vi "Periodic Tasks.vi"(8 "error in":errorcluster) -> ()   [LabVIEW 2016]
doc: "This VI runs in parallel to other tasks. It can contain as many user-defined periodic loops as you need. These can carry out PID or other sorts of timed response."
uses:
  <vilib>/Rock Robotics/WPI/Utilities/WPI_GetSetVariantRefNum.vi
  Robot Global Data.vi
  <vilib>/Rock Robotics/Network Tables/NT Write Number.vi
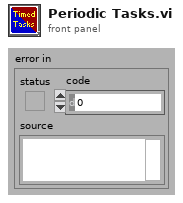
[diagram p1: front panel]
types:
  T1 = typedef "WPI_JoystickDevRef.ctl" = cluster{"Device":T2}
  T2 = typedef "WPI_JoystickDeviceEnum.ctl" = enum16{"USB 0", "USB 1", "USB 2", "USB 3", "USB 4", "USB 5"}
  T3 = typedef "WPI_RobotDriveDevRef.ctl" = cluster{"DevStatus":errorcluster, "Motors[]":T4[], "Square Inputs":bool, "Max Output":dbl}
  T4 = typedef "WPI_MotorControlDeviceRef.ctl" = cluster{"DeviceStatus":errorcluster, "Type":T5, "PWM":cluster{"PWM Channel":T6, "DeadBand":T7}, "CAN":cluster{"Device Number":u8, "SetOutput VI Ref":variant, "GetOutput VI Ref":variant, "Enable VI Ref":variant, "Disable VI Ref":variant, "Data":variant}, "Invert":bool}
  T5 = typedef "WPI_MotorControlType.ctl" = enum16{"PWM", "CAN"}
  T6 = typedef "FPGA_DIOPWMChannel.ctl" = enum8{"PWM 0", "PWM 1", "PWM 2", "PWM 3", "PWM 4", "PWM 5", "PWM 6", "PWM 7", "PWM 8", "PWM 9", "PWM MXP 0", "PWM MXP 1", "PWM MXP 2", "PWM MXP 3", "PWM MXP 4", "PWM MXP 5", "PWM MXP 6", "PWM MXP 7", "PWM MXP 8", "PWM MXP 9", "Invalid"}
  T7 = typedef "WPI_PWMDeadband.ctl" = cluster{"Name":string, "maxPositivePwm":i32, "minPositivePwm":i32, "centerPwm":i32, "maxNegativePwm":i32, "minNegativePwm":i32, "angularRange":u16}
  T8 = typedef "WPI_EncoderDevRef.ctl" = cluster{"DevStatus":errorcluster, "EncoderIndex":T9, "CounterIndex":T10, "DistancePerCount":dbl, "Decoding Type":T11}
  T9 = typedef "FPGA_EncoderIdx.ctl" = enum8{"Enc 0", "Enc 1", "Enc 2", "Enc 3", "Enc 4", "Enc 5", "Enc 6", "Enc 7", "Invalid"}
  T10 = typedef "FPGA_CounterCtrSystemIndex.ctl" = enum8{"Ctr 0", "Ctr 1", "Ctr 2", "Ctr 3", "Ctr 4", "Ctr 5", "Ctr 6", "Ctr 7", "Invalid"}
  T11 = typedef "WPI_EncoderType.ctl" = enum16{"1x", "2x", "4x"}
  T12 = typedef "WPI_ServoDeviceRef.ctl" = cluster{"DeviceStatus":errorcluster, "PWM Channel":T6, "DeadBand":T7}
  T13 = cluster{"JoystickDevRef":T1, "RobotDriveDevRef":T3, "JoystickDevRef":T1}
  T14 = cluster{"Buttons[0]":bool, "Buttons[1]":bool, "Buttons[2]":bool, "Buttons[3]":bool, "Buttons[4]":bool, "Buttons[5]":bool, "Buttons[6]":bool, "Buttons[7]":bool, "Buttons[8]":bool}
  T15 = cluster{"Axes[0]":dbl, "Axes[1]":dbl, "Axes[2]":dbl, "Axes[3]":dbl, "Axes[4]":dbl, "Axes[5]":dbl, "Axes[6]":dbl, "Axes[7]":dbl, "Axes[8]":dbl}
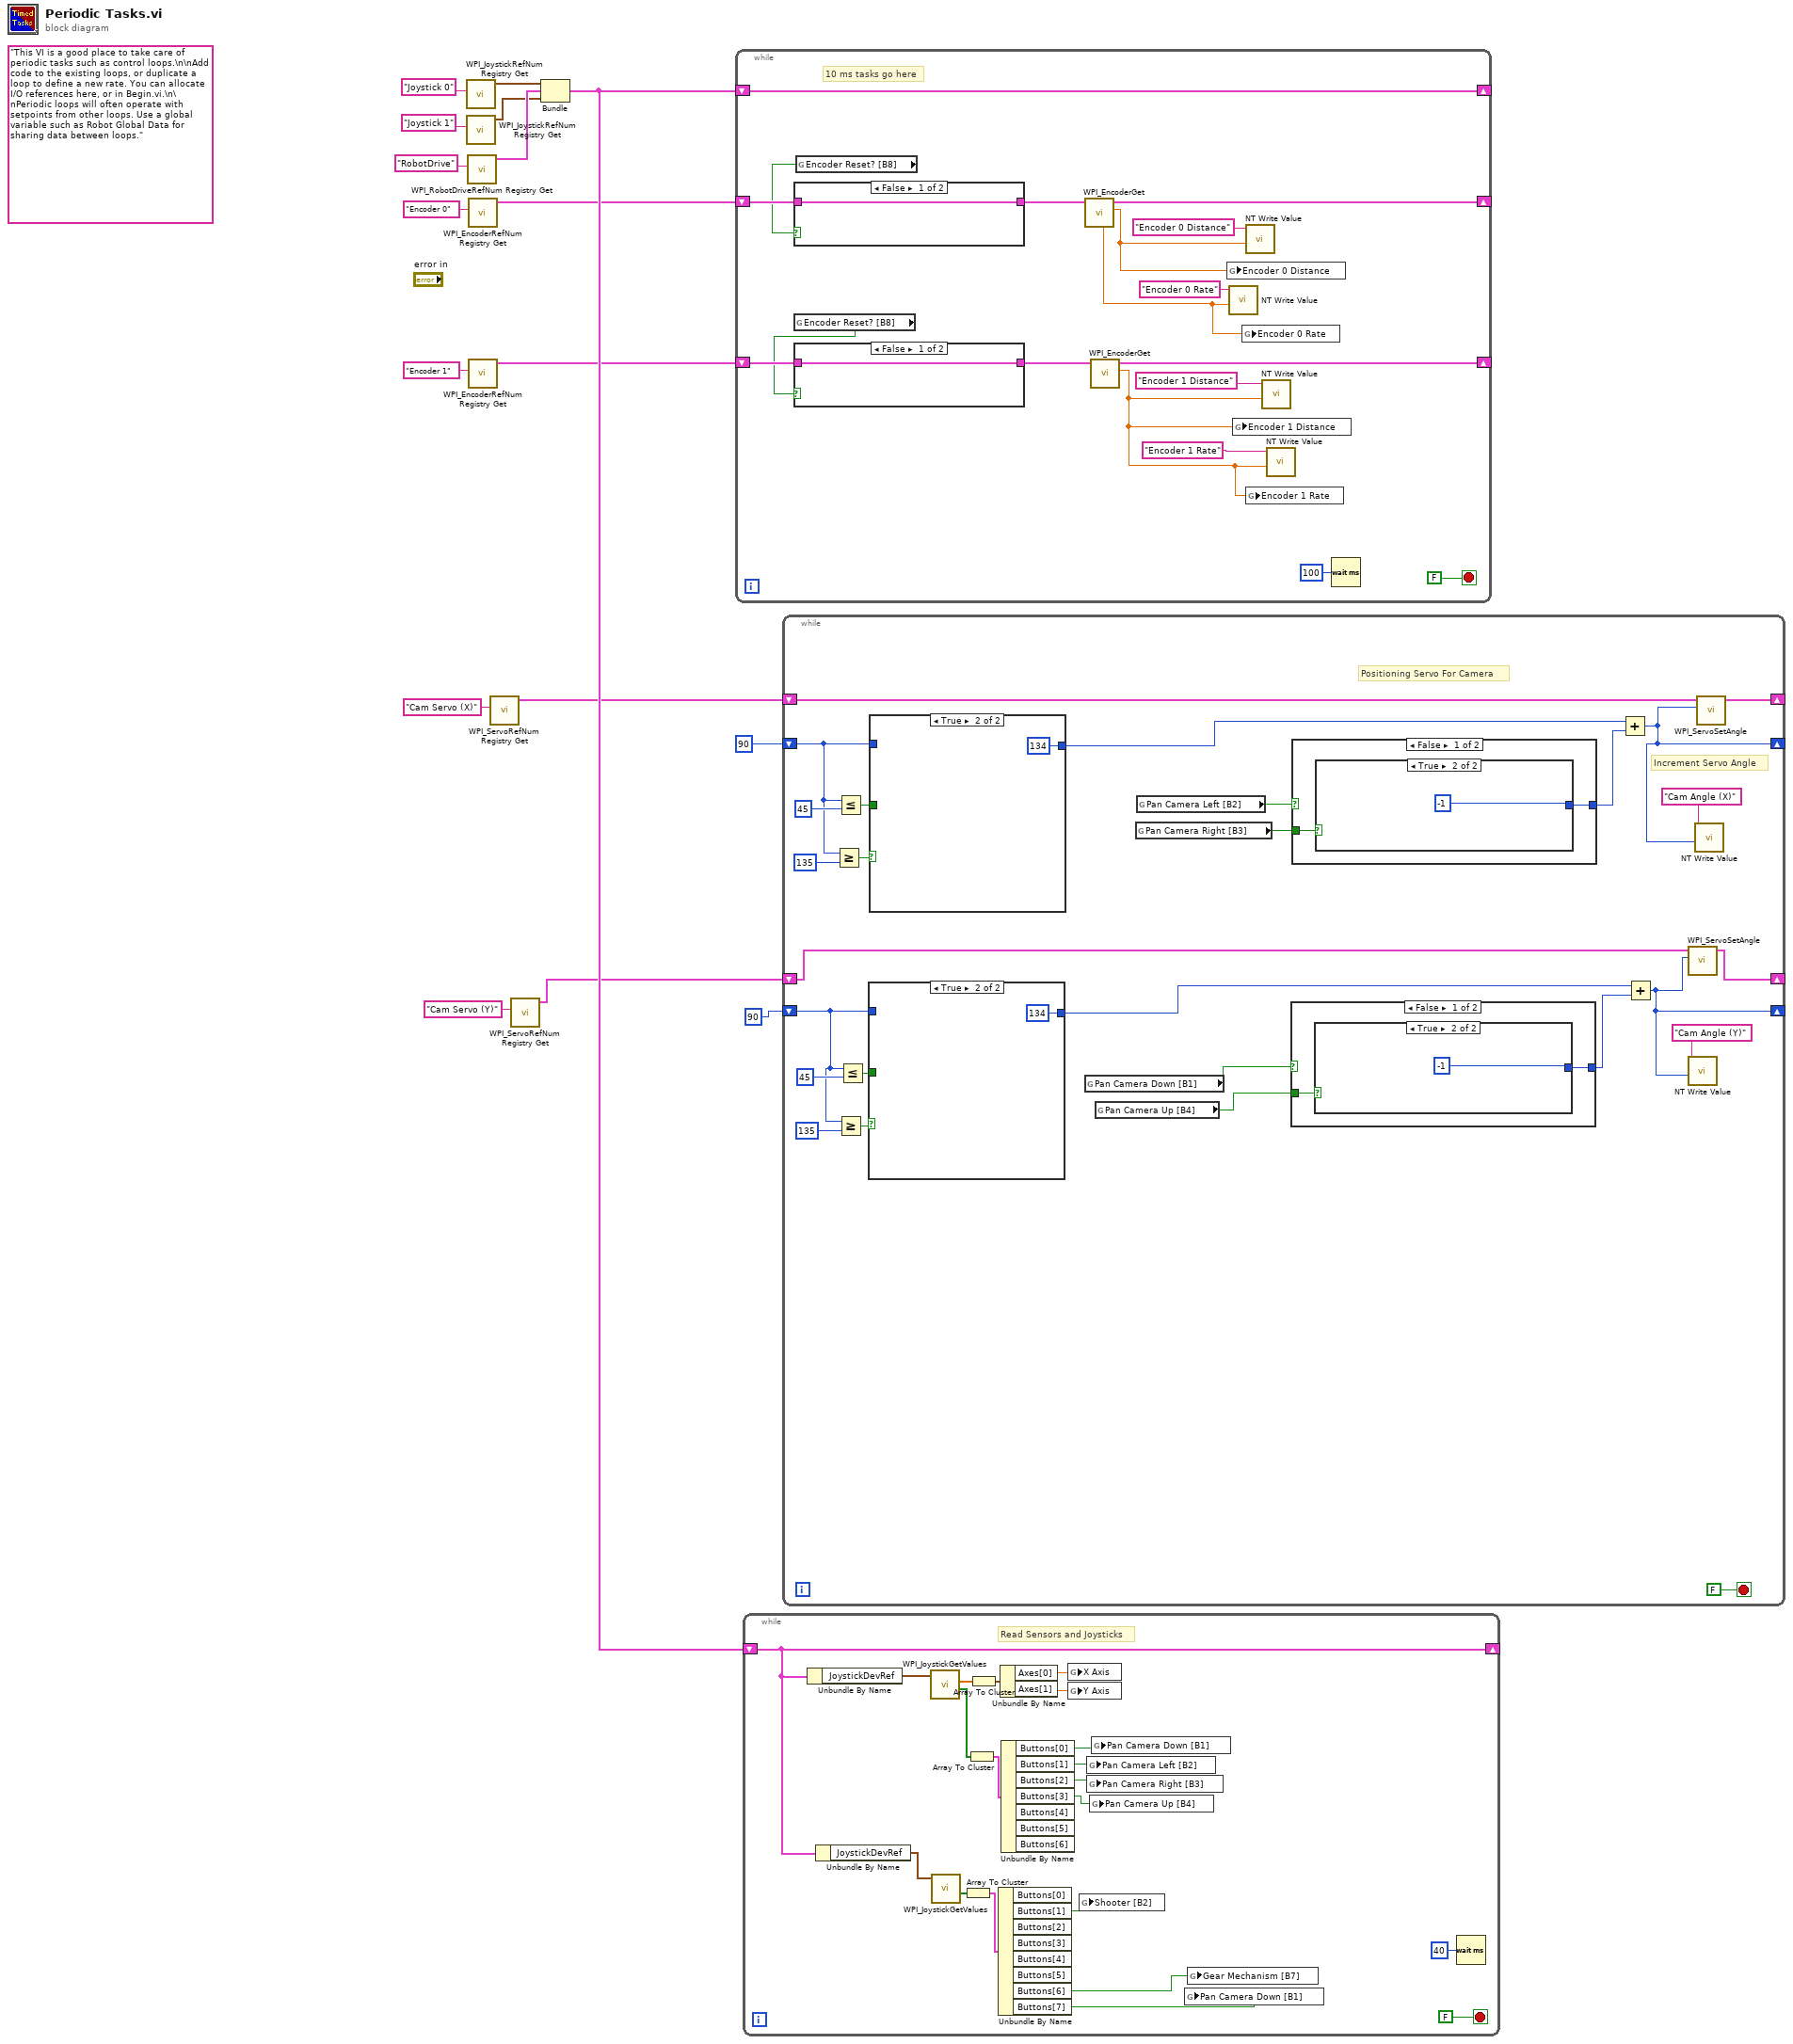
[diagram p0: block diagram]
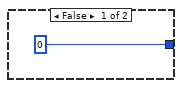
[diagram p2: hidden frame]
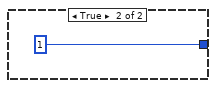
[diagram p3: hidden frame]
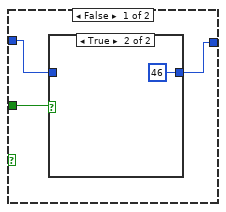
[diagram p4: hidden frame]
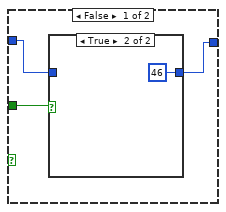
[diagram p6: hidden frame]
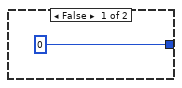
[diagram p8: hidden frame]
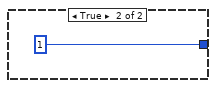
[diagram p9: hidden frame]
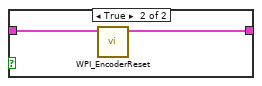
[diagram p10: hidden frame]
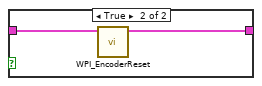
[diagram p11: hidden frame]
diagram:
  (unwired) "This VI is a good place to take care of periodic tasks such as control loops.\n\nAdd code to the existing loops, or duplicate a loop to define a new rate. You can allocate I/O references here, or in Begin.vi.\n\nPeriodic loops will often operate with setpoints from other loops. Use a global variable such as Robot Global Data for sharing data between loops."
  n1 = call <vilib>:"WPI_JoystickRefNum Registry Get.vi"("refnum name"="Joystick 0") -> ("JoystickDevRef"=w15:T1)  [unwired: 1 in, 9 out]
  n2 = call <vilib>:"WPI_JoystickRefNum Registry Get.vi"("refnum name"="Joystick 1") -> ("JoystickDevRef"=w1:T1)  [unwired: 1 in, 9 out]
  n3 = call <vilib>:"WPI_RobotDriveRefNum Registry Get.vi"("refnum name"="RobotDrive") -> ("RobotDriveDevRef"=w14:T3)  [unwired: 1 in, 9 out]
  n4 = call <vilib>:"WPI_EncoderRefNum Registry Get.vi"("refnum name"="Encoder 0") -> ("EncoderDevRef"=w11:T8)  [unwired: 9 in, 1 out]
  n5 = call <vilib>:"WPI_EncoderRefNum Registry Get.vi"("refnum name"="Encoder 1") -> ("EncoderDevRef"=w8:T8)  [unwired: 9 in, 1 out]
  n6 = call <vilib>:"WPI_ServoRefNum Registry Get.vi"("refnum name"="Cam Servo (X)") -> ("ServoDeviceRef"=w5:T12)  [unwired: 9 in, 1 out]
  n7 = call <vilib>:"WPI_ServoRefNum Registry Get.vi"("refnum name"="Cam Servo (Y)") -> ("ServoDeviceRef"=w2:T12)  [unwired: 9 in, 1 out]
  n8 = Bundle("JoystickDevRef"=w15, "RobotDriveDevRef"=w14, "JoystickDevRef"=w1) -> (w13:T13)  [unwired: 1 out]
  n9 = while {
    shift-right: [w33] -> _
    shift-left: w13 -> [w33]
    shift-right: [w27] -> _
    shift-left: w11 -> [w30]
    shift-right: [w23] -> _
    shift-left: w8 -> [w26]
    stop <- FALSE stop-if-true
    # "10 ms tasks go here"
    n10 = global read "Robot Global Data.vi" "Encoder Reset? [B8]"() -> (w25:bool)
    n11 = case shown="False" w25 {
      tunnel: w26 -> [w36 w38]
      tunnel: [w36 w37] -> w24
      frame False {
      }
      frame True {
        n12 = call <vilib>:"WPI_EncoderReset.vi"("EncoderDevRef"=w38) -> ("EncoderDevRef"=w37:T8)  [unwired: 9 in, 1 out]
      }
    }
    n13 = global read "Robot Global Data.vi" "Encoder Reset? [B8]"() -> (w28:bool)
    n14 = case shown="False" w28 {
      tunnel: w30 -> [w39 w41]
      tunnel: [w39 w40] -> w29
      frame False {
      }
      frame True {
        n15 = call <vilib>:"WPI_EncoderReset.vi"("EncoderDevRef"=w41) -> ("EncoderDevRef"=w40:T8)  [unwired: 9 in, 1 out]
      }
    }
    n16 = call <vilib>:"WPI_EncoderGet.vi"("EncoderDevRef"=w29) -> ("Distance"=w32:dbl, "EncoderDevRef"=w27:T8, "Rate"=w19:dbl)  [unwired: 5 in, 3 out]
    n17 = call <vilib>:"WPI_EncoderGet.vi"("EncoderDevRef"=w24) -> ("Distance"=w18:dbl, "EncoderDevRef"=w23:T8)  [unwired: 5 in, 4 out]
    n18 = global write "Robot Global Data.vi" "Encoder 0 Distance"(w32) -> ()
    n19 = call-poly <vilib>:"NT Write Value.vi"("Numeric"=w19, "Name"="Encoder 0 Rate") -> ()  [unwired: 9 in, 1 out]
    n20 = global write "Robot Global Data.vi" "Encoder 1 Distance"(w18) -> ()
    n21 = global write "Robot Global Data.vi" "Encoder 0 Rate"(w19) -> ()
    n22 = call-poly <vilib>:"NT Write Value.vi"("Numeric"=w32, "Name"="Encoder 0 Distance") -> ()  [unwired: 9 in, 1 out]
    n23 = global write "Robot Global Data.vi" "Encoder 1 Rate"(w18) -> ()
    n24 = call-poly <vilib>:"NT Write Value.vi"("Numeric"=w18, "Name"="Encoder 1 Distance") -> ()  [unwired: 9 in, 1 out]
    n25 = call-poly <vilib>:"NT Write Value.vi"("Numeric"=w18, "Name"="Encoder 1 Rate") -> ()  [unwired: 9 in, 1 out]
    n26 = Wait (ms)(milliseconds to wait=u32 100) -> ()  [unwired: 1 out]
  }
  n27 = while {
    shift-right: [w44] -> _
    shift-left: w13 -> [w44]
    stop <- FALSE stop-if-true
    # "Read Sensors and Joysticks"
    n28 = Unbundle By Name(w44) -> ("JoystickDevRef"=w53:T1)
    n29 = Unbundle By Name(w44) -> ("JoystickDevRef"=w43:T1)
    n30 = call <vilib>:"WPI_JoystickGetValues.vi"("JoystickDevRef"=w53) -> ("Buttons"=w49:bool[], "Axes"=w58:dbl[])  [unwired: 6 in, 3 out]
    n31 = call <vilib>:"WPI_JoystickGetValues.vi"("JoystickDevRef"=w43) -> ("Buttons"=w54:bool[])  [unwired: 6 in, 4 out]
    n32 = Array To Cluster(array=w54) -> (cluster=w55:T14)
    n33 = Array To Cluster(array=w49) -> (cluster=w50:T14)
    n34 = Array To Cluster(array=w58) -> (cluster=w59:T15)
    n35 = Unbundle By Name(w55) -> ("Buttons[1]"=w52:bool, "Buttons[6]"=w42:bool, "Buttons[7]"=w51:bool)  [unwired: 5 out]
    n36 = Unbundle By Name(w59) -> ("Axes[0]"=w57:dbl, "Axes[1]"=w56:dbl)
    n37 = Unbundle By Name(w50) -> ("Buttons[0]"=w45:bool, "Buttons[1]"=w48:bool, "Buttons[2]"=w47:bool, "Buttons[3]"=w46:bool)  [unwired: 3 out]
    n38 = global write "Robot Global Data.vi" "X Axis"(w57) -> ()
    n39 = global write "Robot Global Data.vi" "Y Axis"(w56) -> ()
    n40 = global write "Robot Global Data.vi" "Shooter [B2]"(w52) -> ()
    n41 = global write "Robot Global Data.vi" "Pan Camera Left [B2]"(w48) -> ()
    n42 = global write "Robot Global Data.vi" "Pan Camera Right [B3]"(w47) -> ()
    n43 = global write "Robot Global Data.vi" "Pan Camera Up [B4]"(w46) -> ()
    n44 = global write "Robot Global Data.vi" "Pan Camera Down [B1]"(w45) -> ()
    n45 = global write "Robot Global Data.vi" "Pan Camera Down [B1]"(w51) -> ()
    n46 = global write "Robot Global Data.vi" "Gear Mechanism [B7]"(w42) -> ()
    n47 = Wait (ms)(milliseconds to wait=u32 40) -> ()  [unwired: 1 out]
  }
  n48 = while {
    shift-right: [w86] -> _
    shift-left: w5 -> [w87]
    shift-right: [w76] -> _
    shift-left: 90 -> [w79]
    shift-right: [w64] -> _
    shift-left: 90 -> [w70]
    shift-right: [w62] -> _
    shift-left: w2 -> [w63]
    stop <- FALSE stop-if-true
    # "Increment Servo Angle"
    # "Positioning Servo For Camera"
    n49 = Greater Or Equal?(x=w79, y=135) -> (x >= y?=w78:bool)
    n50 = Less Or Equal?(x=w79, y=45) -> (x <= y?=w77:bool)
    n51 = Greater Or Equal?(x=w70, y=135) -> (x >= y?=w72:bool)
    n52 = Less Or Equal?(x=w70, y=45) -> (x <= y?=w71:bool)
    n53 = case shown="True" w72 {
      tunnel: w70 -> [w96 _]
      tunnel: [w95 134] -> w67
      tunnel: w71 -> [w94 _]
      frame False {
        n54 = case shown="True" w94 {
          tunnel: w96 -> [w97 _]
          tunnel: [w97 46] -> w95
          frame False {
          }
          frame True {
          }
        }
      }
      frame True {
      }
    }
    n55 = case shown="True" w78 {
      tunnel: w79 -> [w102 _]
      tunnel: [w101 134] -> w82
      tunnel: w77 -> [w100 _]
      frame False {
        n56 = case shown="True" w100 {
          tunnel: w102 -> [w103 _]
          tunnel: [w103 46] -> w101
          frame False {
          }
          frame True {
          }
        }
      }
      frame True {
      }
    }
    n57 = global read "Robot Global Data.vi" "Pan Camera Down [B1]"() -> (w69:bool)
    n58 = global read "Robot Global Data.vi" "Pan Camera Up [B4]"() -> (w68:bool)
    n59 = global read "Robot Global Data.vi" "Pan Camera Right [B3]"() -> (w84:bool)
    n60 = global read "Robot Global Data.vi" "Pan Camera Left [B2]"() -> (w83:bool)
    n61 = case shown="False" w69 {
      tunnel: [w90 1] -> w66
      tunnel: w68 -> [w89 _]
      frame False {
        n62 = case shown="True" w89 {
          tunnel: [0 -1] -> w90
          frame False {
          }
          frame True {
          }
        }
      }
      frame True {
      }
    }
    n63 = case shown="False" w83 {
      tunnel: [w107 1] -> w85
      tunnel: w84 -> [w106 _]
      frame False {
        n64 = case shown="True" w106 {
          tunnel: [0 -1] -> w107
          frame False {
          }
          frame True {
          }
        }
      }
      frame True {
      }
    }
    n65 = Add(x=w82, y=w85) -> (x+y=w76:i32)
    n66 = Add(x=w67, y=w66) -> (x+y=w64:i32)
    n67 = call <vilib>:"WPI_ServoSetAngle.vi"("Angle"=w64, "ServoDeviceRef"=w63) -> ("ServoDeviceRef"=w62:T12)  [unwired: 8 in, 1 out]
    n68 = call-poly <vilib>:"NT Write Value.vi"("Numeric"=w64, "Name"="Cam Angle (Y)") -> ()  [unwired: 9 in, 1 out]
    n69 = call-poly <vilib>:"NT Write Value.vi"("Numeric"=w76, "Name"="Cam Angle (X)") -> ()  [unwired: 9 in, 1 out]
    n70 = call <vilib>:"WPI_ServoSetAngle.vi"("Angle"=w76, "ServoDeviceRef"=w87) -> ("ServoDeviceRef"=w86:T12)  [unwired: 8 in, 1 out]
  }
